vi "Read Local Repository.vi"(11 "Artifactory in":refnum<class "Artifactory.lvclass">) -> (2 "Local Repository":path, 3 "Artifactory out":refnum<class "Artifactory.lvclass">)   [LabVIEW 2021, in "Artifactory.lvclass"]
uses:
  Artifactory.lvclass
  Artifactory.lvclass/Artifactory.ctl
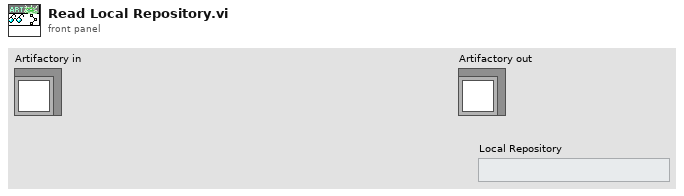
[diagram p1: front panel]
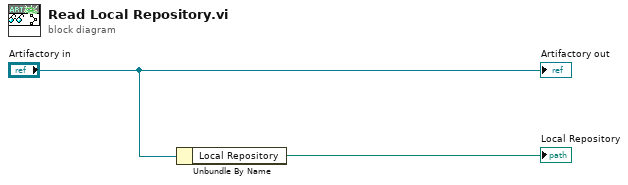
[diagram p0: block diagram]
diagram:
  n1 = Unbundle By Name("Artifactory in") -> ("Local Repository"=→"Local Repository":path)
  "Artifactory out" <- "Artifactory in"
